vi "disable debugging.vi"(10 "parameters":variant[](array[variant]), 11 "vis":refnum<vi>[](array[refnum])) -> (0 "error report":errorcluster[](array[cluster]))   [LabVIEW 2013]
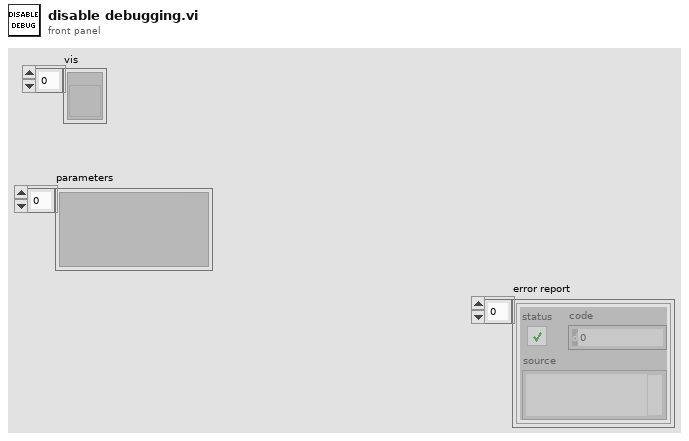
[diagram p1: front panel]
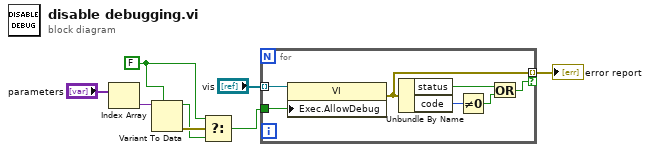
[diagram p0: block diagram]
diagram:
  w3 = FALSE
  n1 = Index Array(array="parameters") -> (element=w5:variant)  [unwired: 1 in]
  n2 = Variant To Data(type=w3, Variant=w5) -> (data=w2:bool, error out=w4:errorcluster)  [unwired: 1 in]
  n3 = Select(t=w3, s=w4, f=w2) -> (s? t:f=w1:bool)
  n4 = for {
    tunnel: "vis" -> [w15] mode=indexing
    tunnel: [w11] -> w7 mode=indexing if=w10
    tunnel: w1 -> [w9]
    n5 = property class="VI"(reference=w15, "Exec.AllowDebug"=w9) -> (error out=w11:errorcluster)  [unwired: 1 in, 1 out]
    n6 = Unbundle By Name(w11) -> ("status"=w14:bool, "code"=w13:i32)
    n7 = Not Equal To 0?(x=w13) -> (x != 0?=w12:bool)
    n8 = Or(x=w14, y=w12) -> (x .or. y?=w10:bool)
  }
  "error report" <- w7
